vi "mClampAxon1D.vi"() -> ()   [LabVIEW 2012]
uses:
  <vilib>/DAQmx/write.llb/DAQmx Write (Analog Wfm 1Chan NSamp).vi
  <vilib>/DAQmx/read.llb/DAQmx Read (Analog 1D Wfm NChan NSamp).vi
  <vilib>/DAQmx/create/channels.llb/DAQmx Create Channel (AI-Voltage-Basic).vi
  <vilib>/DAQmx/configure/timing.llb/DAQmx Timing (Sample Clock).vi
  <vilib>/DAQmx/create/channels.llb/DAQmx Create Channel (AO-Voltage-Basic).vi
  <vilib>/DAQmx/miscellaneous.llb/DAQmx Fill In Error Info.vi
  <vilib>/Analysis/baseanly.llb/Mean (DBL).vi
  <vilib>/Analysis/NI_AALBase.lvlib
  <vilib>/ptbypt/NI_PtbyPt.lvlib
  <vilib>/Analysis/NI_AALPro.lvlib
panel:
  in  "Upper Cut-Off":dbl=250.0
  in  "Lower Cut-Off":dbl=0.0001
  in  "duration(msec)":u32=20 caption="duration (msec)"
  in  "mfactor":dbl=50.0
  in  "Sound":bool
  in  "Gain (b)":bool=TRUE
  out "reversed array":i32[](array[numeric])
  out "R Graph":dynamicdata(graph)
  out "refresh":bool
  in  "Amplitude (pA)":dbl=10.0
  out "Raw Voltage":dynamicdata(graph)
  in  "Voltage Clamp":bool=TRUE
  out "Resistance\n (MOhm)":dbl
  out "Off":bool
  out "On":bool
  in  "Amplitude (mV)":dbl=10.0
  in  "R test":bool
  in  "Off Time (msec)":u32=100
  in  "On Time (msec)":u32=50
  in  "stop":bool
  # "Amplifier Settings"
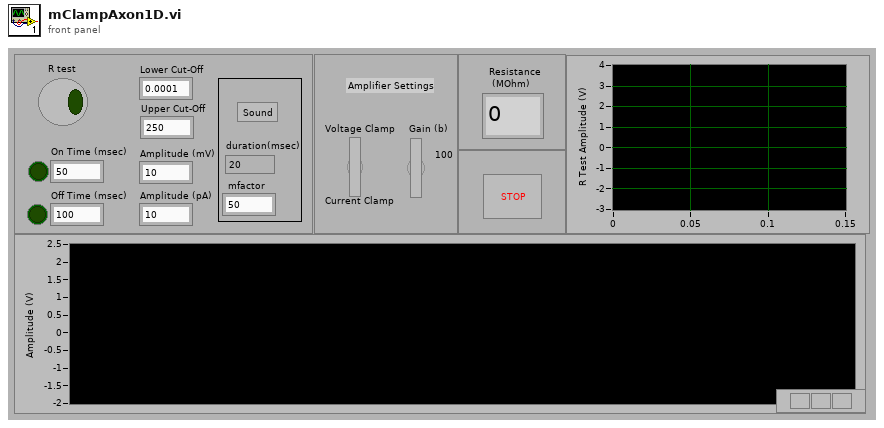
[diagram p1: front panel]
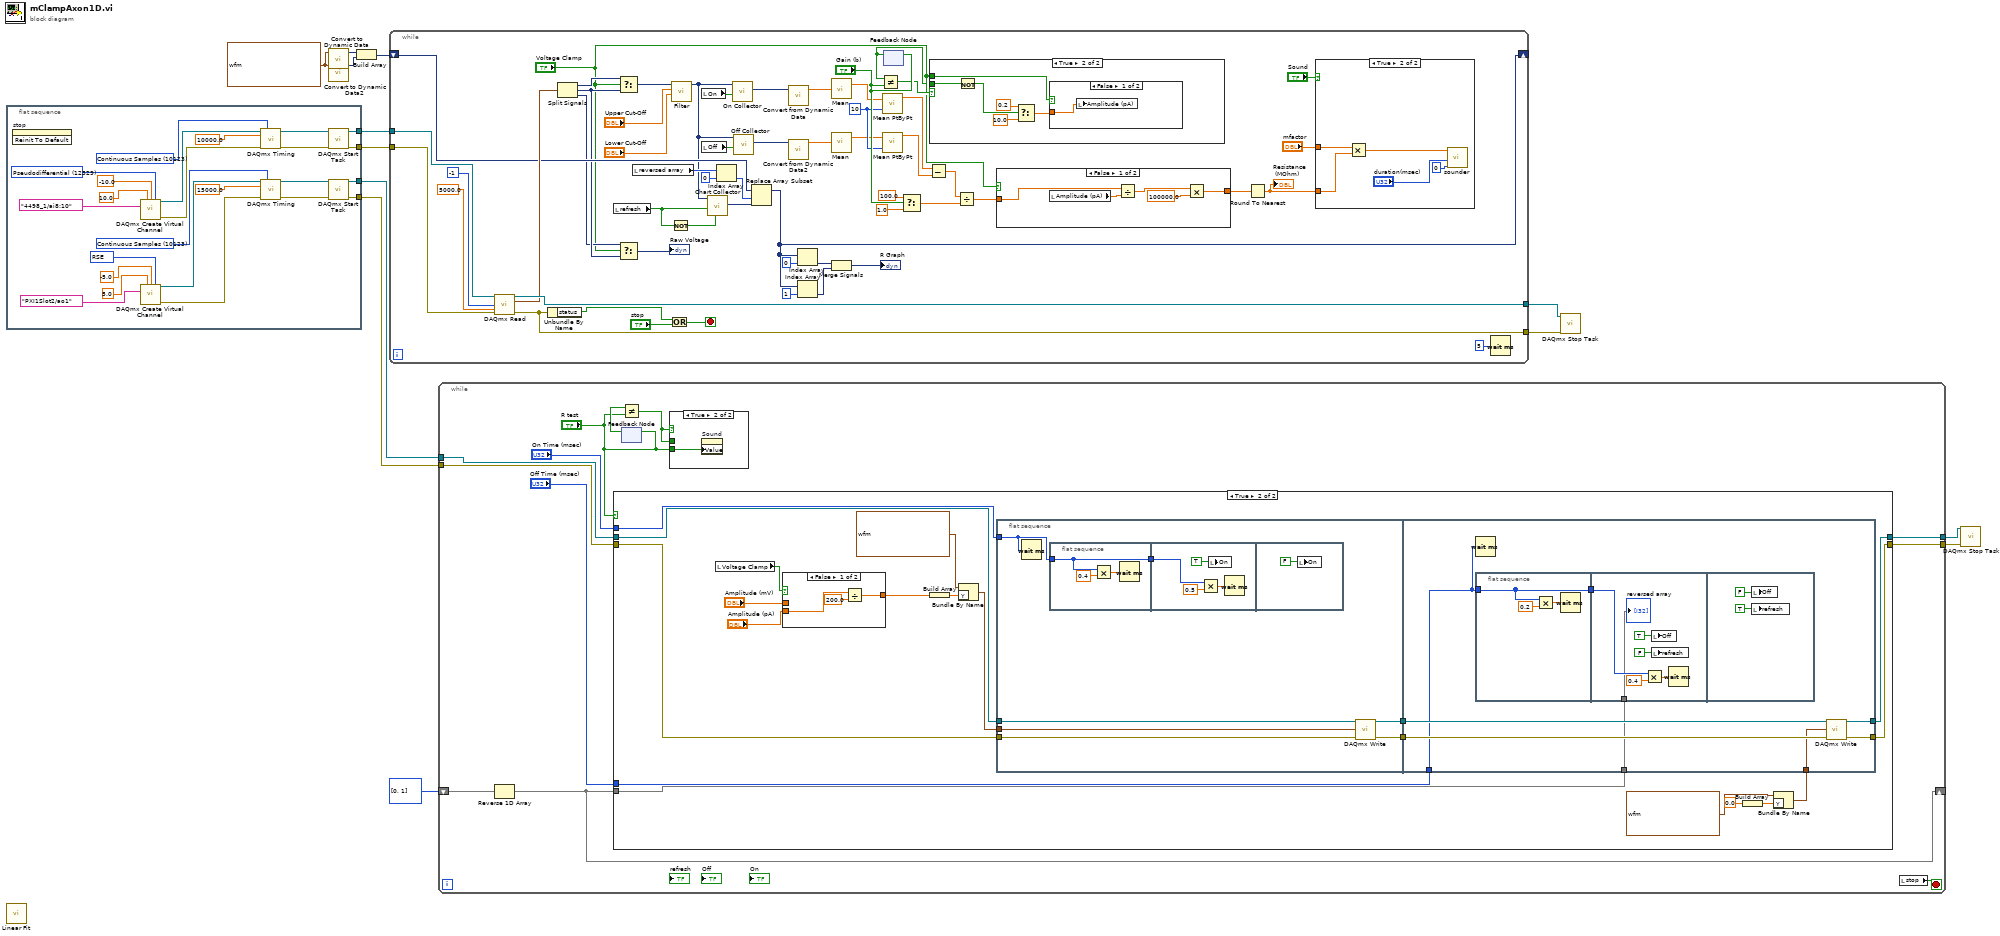
[diagram p0: block diagram]
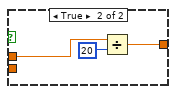
[diagram p4: hidden frame]
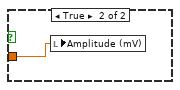
[diagram p6: hidden frame]
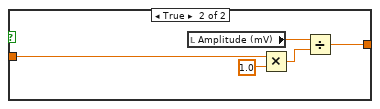
[diagram p8: hidden frame]
diagram:
  w5 = waveform(dbl) {"t0"=timestamp(0 s since 1904-01-01), "dt"=1.0, "Y"=[]} ("Waveform")
  n1 = flat-sequence {
    tunnel: [w29] -> w13
    tunnel: [w28] -> w12
    tunnel: [w15] -> w9
    tunnel: [w14] -> w8
    frame #0 {
      w25 = 10083 items=["default"=-1, "RSE"=10083, "NRSE"=10078, "Differential"=10106, "Pseudodifferential"=12529] ("input terminal configuration")
      w21 = 10123 items=["Finite Samples"=10178, "Continuous Samples"=10123, "Hardware Timed Single Point"=12522] ("sample mode")
      w26 = 12529 items=["default"=-1, "RSE"=10083, "NRSE"=10078, "Differential"=10106, "Pseudodifferential"=12529] ("input terminal configuration")
      w33 = 10123 items=["Finite Samples"=10178, "Continuous Samples"=10123, "Hardware Timed Single Point"=12522] ("sample mode")
      n2 = invoke on="stop" class="Bool (strict)" method="Reinit To Default"() -> ()  [unwired: 3 in, 3 out]
      n3 = call-poly <vilib>:"DAQmx Create Virtual Channel.vi"("maximum value"=10.0, "minimum value"=-10.0, "input terminal configuration"=w26, "physical channels"=tag "4498_1/ai8:10") -> ("task out"=w35:refnum<k21>, "error out"=w34:errorcluster)  [unwired: 10 in]
      n4 = call-poly <vilib>:"DAQmx Create Virtual Channel.vi"("maximum value"=5.0, "minimum value"=-5.0, "output terminal configuration"=w25, "physical channels"=tag "PXI1Slot2/ao1" ("physical channels 2")) -> ("task out"=w19:refnum<k21>, "error out"=w20:errorcluster)  [unwired: 10 in]
      n5 = call-poly <vilib>:"DAQmx Timing.vi"("task/channels in"=w35, "sample mode"=w33, "rate"=10000.0, "error in"=w34) -> ("task out"=w37:refnum<k21>, "error out"=w36:errorcluster)  [unwired: 10 in]
      n6 = call-poly <vilib>:"DAQmx Timing.vi"("task/channels in"=w19, "sample mode"=w21, "rate"=15000.0, "error in"=w20) -> ("task out"=w17:refnum<k21>, "error out"=w18:errorcluster)  [unwired: 10 in]
      n7 = call <vilib>:"DAQmx Start Task.vi"("task/channels in"=w37, "error in"=w36) -> ("task out"=w29:refnum<k21>, "error out"=w28:errorcluster)  [unwired: 12 in]
      n8 = call <vilib>:"DAQmx Start Task.vi"("task/channels in"=w17, "error in"=w18) -> ("task out"=w15:refnum<k21>, "error out"=w14:errorcluster)  [unwired: 12 in]
    }
  }
  n9 = call <vilib>:"Linear Fit.vi"() -> ()  [unwired: 11 in, 5 out]
  n10 = call "Convert to Dynamic Data"("Waveform"=w5) -> ("Dynamic Data Type"=w3:dynamicdata)  [unwired: 3 in]
  n11 = call "Convert to Dynamic Data2"("Waveform"=w5) -> ("Dynamic Data Type"=w4:dynamicdata)  [unwired: 3 in]
  n12 = Build Array(w3, w4) -> (w2:dynamicdata[])
  n13 = while {
    tunnel: w13 -> [w91]
    tunnel: w12 -> [w90]
    tunnel: [w89] -> w7
    tunnel: [w74] -> w6
    shift-right: [w76] -> _
    shift-left: w2 -> [w80]
    stop <- w71 stop-if-true
    w43 = 10 ("sample length")
    n14 = call-poly <vilib>:"DAQmx Read.vi"("task/channels in"=w91, "number of samples per channel"=-1, "timeout"=5000.0, "error in"=w90) -> ("task out"=w89:refnum<k21>, "data"=w88:waveform(dbl)[], "error out"=w74:errorcluster)  [unwired: 9 in]
    n15 = Unbundle By Name(w74) -> ("status"=w73:bool)
    n16 = Split Signals(w88) -> (w70:dynamicdata, w60:dynamicdata, w59:dynamicdata)  [unwired: 3 in]
    n17 = local read "refresh"() -> (w87:bool)
    n18 = Select(t=w70, s="Voltage Clamp", f=w60) -> (s? t:f=w54:dynamicdata)
    n19 = Select(t=w59, s="Voltage Clamp", f=w60) -> (s? t:f=→"Raw Voltage":dynamicdata)
    n20 = local read "reversed array"() -> (w79:i32[])
    n21 = Or(x=w73, y="stop") -> (x .or. y?=w71:bool)
    n22 = Not(x=w87) -> (.not. x?=w86:bool)
    n23 = call "Filter"("Lower Cut-Off"="Lower Cut-Off", "Upper Cut-Off"="Upper Cut-Off", "Signal"=w54) -> ("Filtered Signal"=w44:dynamicdata)  [unwired: 7 in, 1 out]
    n24 = local read "On"() -> (w50:bool)
    n25 = local read "Off"() -> (w49:bool)
    n26 = call "Chart Collector"("Reset"=w86, "Enable"=w87, "Signals"=w44) -> ("Collected Signals"=w85:dynamicdata)  [unwired: 7 in, 1 out]
    n27 = Index Array(array=w79, index=0) -> (element=w77:i32)
    n28 = call "On Collector"("Enable"=w50, "Signals"=w44) -> ("Collected Signals"=w48:dynamicdata)  [unwired: 8 in, 1 out]
    n29 = call "Off Collector"("Enable"=w49, "Signals"=w44) -> ("Collected Signals"=w46:dynamicdata)  [unwired: 8 in, 1 out]
    n30 = Replace Array Subset(array=w80, new element=w85, index=w77) -> (w76:dynamicdata[])
    n31 = call "Convert from Dynamic Data"("Dynamic Data Type"=w48) -> ("Array"=w47:dbl[])  [unwired: 3 in]
    n32 = call "Convert from Dynamic Data2"("Dynamic Data Type"=w46) -> ("Array"=w45:dbl[])  [unwired: 3 in]
    n33 = Index Array(array=w76, index=0) -> (element=w84:dynamicdata)
    n34 = Index Array(array=w76, index=1) -> (element=w83:dynamicdata)
    n35 = call-poly <vilib>:"Mean.vi"("X"=w47) -> ("mean"=w42:dbl)  [unwired: 1 out]
    n36 = call-poly <vilib>:"Mean.vi"("X"=w45) -> ("mean"=w40:dbl)  [unwired: 1 out]
    n37 = Merge Signals(w84, w83) -> (→"R Graph":dynamicdata)
    n38 = call <vilib>:"Mean PtByPt.vi"("x"=w42, "sample length"=w43) -> ("mean"=w41:dbl)  [unwired: 2 in, 1 out]
    n39 = call <vilib>:"Mean PtByPt.vi"("x"=w40, "sample length"=w43) -> ("mean"=w39:dbl)  [unwired: 2 in, 1 out]
    n40 = feedback-in #1("Gain (b)") -> ()
    n41 = feedback #1() -> (w55:bool)  [unwired: 1 in]
    n42 = Not Equal?(x=w55, y="Gain (b)") -> (x != y?=w57:bool)
    n43 = Select(t=100.0, s="Gain (b)", f=1.0) -> (s? t:f=w66:dbl)
    n44 = Subtract(x=w41, y=w39) -> (x-y=w65:dbl)
    n45 = case shown="True" w57 {
      tunnel: w55 -> [_ w95]
      tunnel: "Voltage Clamp" -> [_ w96]
      frame False {
      }
      frame True {
        n46 = Not(x=w95) -> (.not. x?=w94:bool)
        n47 = Select(t=0.2, s=w94, f=10.0) -> (s? t:f=w97:dbl)
        n48 = case shown="False" w96 {
          tunnel: w97 -> [w100 w101]
          frame False {
            n49 = local write "Amplitude (pA)"(w100) -> ()
          }
          frame True {
            n50 = local write "Amplitude (mV)"(w101) -> ()
          }
        }
      }
    }
    n51 = Divide(x=w65, y=w66) -> (x/y=w67:dbl)
    n52 = case shown="False" "Voltage Clamp" {
      tunnel: w67 -> [w108 w113]
      tunnel: [w107 w112] -> w62
      frame False {
        n53 = local read "Amplitude (pA)"() -> (w109:dbl)
        n54 = Divide(x=w108, y=w109) -> (x/y=w110:dbl)
        n55 = Multiply(x=w110, y=100000.0) -> (x*y=w107:dbl)
      }
      frame True {
        n56 = local read "Amplitude (mV)"() -> (w116:dbl)
        n57 = Multiply(x=w113, y=1.0) -> (x*y=w115:dbl)
        n58 = Divide(x=w116, y=w115) -> (x/y=w112:dbl)
      }
    }
    n59 = Round To Nearest(number=w62) -> (nearest integer value=w61:dbl)
    "Resistance\n (MOhm)" <- w61
    n60 = case shown="True" "Sound" {
      tunnel: "mfactor" -> [_ w104]
      tunnel: w61 -> [_ w103]
      frame False {
      }
      frame True {
        n61 = Multiply(x=w104, y=w103) -> (x*y=w105:dbl)
        n62 = call "sounder.vi"("milliseconds to wait"=u32 0, "duration (msec)"="duration(msec)", "frequency (Hz)"=w105) -> ()  [unwired: 9 in]
      }
    }
    n63 = Wait (ms)(milliseconds to wait=u32 5) -> ()  [unwired: 1 out]
  }
  n64 = while {
    tunnel: [w127] -> w11
    tunnel: [w122] -> w10
    tunnel: w9 -> [w124]
    tunnel: w8 -> [w123]
    shift-right: [w120] -> _
    shift-left: i32[] [0, 1] -> [w121]
    stop <- w128 stop-if-true
    n65 = Reverse 1D Array(array=w121) -> (reversed array=w120:i32[])
    n66 = case shown="True" "R test" {
      tunnel: [w131 w149] -> w127
      tunnel: "On Time (msec)" -> [_ w148]
      tunnel: "Off Time (msec)" -> [_ w147]
      tunnel: w124 -> [w131 w146]
      tunnel: w123 -> [w130 w145]
      tunnel: [w130 w144] -> w122
      tunnel: w120 -> [_ w143]
      frame False {
      }
      frame True {
        n67 = local read "Voltage Clamp"() -> (w141:bool)
        n68 = case shown="False" w141 {
          tunnel: [w152 w155] -> w142
          tunnel: "Amplitude (mV)" -> [_ w157]
          tunnel: "Amplitude (pA)" -> [w154 _]
          frame False {
            n69 = Divide(x=w154, y=200.0) -> (x/y=w152:dbl)
          }
          frame True {
            n70 = Divide(x=w157, y=20) -> (x/y=w155:dbl)
          }
        }
        n71 = Build Array(w142) -> (w137:dbl[])
        n72 = Bundle By Name(cluster=waveform(dbl) {"t0"=timestamp(0 s since 1904-01-01), "dt"=1.0, "Y"=[]} ("Waveform"), "Y"=w137) -> (w136:waveform(dbl))
        n73 = flat-sequence {
          tunnel: [w164] -> w151
          tunnel: [w163] -> w150
          tunnel: w148 -> [w161]
          tunnel: w146 -> [w160]
          tunnel: w145 -> [w159]
          tunnel: w136 -> [w158]
          tunnel: w151 -> [w180]
          tunnel: w150 -> [w179]
          tunnel: [w178] -> w149
          tunnel: [w177] -> w144
          tunnel: w147 -> [w175]
          tunnel: w143 -> [w174]
          tunnel: w132 -> [w173]
          frame #0 {
            n74 = Wait (ms)(milliseconds to wait=w161) -> ()  [unwired: 1 out]
            n75 = flat-sequence {
              tunnel: w161 -> [w165]
              tunnel: [w165] -> w162
              tunnel: w162 -> [w168]
              frame #0 {
                n76 = Multiply(x=w165, y=0.4) -> (x*y=w167:dbl)
                n77 = Wait (ms)(milliseconds to wait=w167) -> ()  [unwired: 1 out]
              }
              frame #1 {
                n78 = Multiply(x=w168, y=0.5) -> (x*y=w169:dbl)
                n79 = local write "On"(TRUE) -> ()
                n80 = Wait (ms)(milliseconds to wait=w169) -> ()  [unwired: 1 out]
              }
              frame #2 {
                n81 = local write "On"(FALSE ("Detect")) -> ()
              }
            }
            n82 = call-poly <vilib>:"DAQmx Write.vi"("task/channels in"=w160, "data"=w158, "error in"=w159) -> ("task out"=w164:refnum<k21>, "error out"=w163:errorcluster)  [unwired: 10 in, 1 out]
          }
          frame #1 {
            n83 = Wait (ms)(milliseconds to wait=w175) -> ()  [unwired: 1 out]
            n84 = flat-sequence {
              tunnel: w175 -> [w181]
              tunnel: [w181] -> w176
              tunnel: w176 -> [w186]
              tunnel: w174 -> [w184]
              frame #0 {
                n85 = Multiply(x=w181, y=0.2) -> (x*y=w183:dbl)
                n86 = Wait (ms)(milliseconds to wait=w183) -> ()  [unwired: 1 out]
              }
              frame #1 {
                n87 = Multiply(x=w186, y=0.4) -> (x*y=w187:dbl)
                n88 = local write "Off"(TRUE) -> ()
                n89 = local write "refresh"(FALSE ("refresh")) -> ()
                n90 = Wait (ms)(milliseconds to wait=w187) -> ()  [unwired: 1 out]
                "reversed array" <- w184
              }
              frame #2 {
                n91 = local write "Off"(FALSE ("Detect")) -> ()
                n92 = local write "refresh"(TRUE ("refresh")) -> ()
              }
            }
            n93 = call-poly <vilib>:"DAQmx Write.vi"("task/channels in"=w180, "data"=w173, "error in"=w179) -> ("task out"=w178:refnum<k21>, "error out"=w177:errorcluster)  [unwired: 10 in, 1 out]
          }
        }
        n94 = Build Array(0.0) -> (w134:dbl[])
        n95 = Bundle By Name(cluster=waveform(dbl) {"t0"=timestamp(0 s since 1904-01-01), "dt"=1.0, "Y"=[]} ("Waveform"), "Y"=w134) -> (w132:waveform(dbl))
      }
    }
    n96 = feedback-in #2("R test") -> ()
    n97 = feedback #2() -> (w119:bool)  [unwired: 1 in]
    n98 = Not Equal?(x=w119, y="R test") -> (x != y?=w118:bool)
    n99 = case shown="True" w118 {
      tunnel: w118 -> [_ _]
      tunnel: "R test" -> [_ w129]
      frame False {
      }
      frame True {
        n100 = property on="Sound" class="Bool (strict)"("Value"=w129) -> ()  [unwired: 2 in, 2 out]
      }
    }
    n101 = local read "stop"() -> (w128:bool)
  }
  n102 = call <vilib>:"DAQmx Stop Task.vi"("task/channels in"=w7, "error in"=w6) -> ()  [unwired: 12 in, 2 out]
  n103 = call <vilib>:"DAQmx Stop Task.vi"("task/channels in"=w11, "error in"=w10) -> ()  [unwired: 12 in, 2 out]
